vi "fWrite Binary.vi"(8 "error in":errorcluster, 9 "Samples per data chunk":u32, 10 "array":i16[](array[numeric]), 11 "refnum in":refnum<file>) -> (0 "error out":errorcluster, 3 "refnum out":refnum<file>, 5 "Data good?":bool)   [LabVIEW 2012]
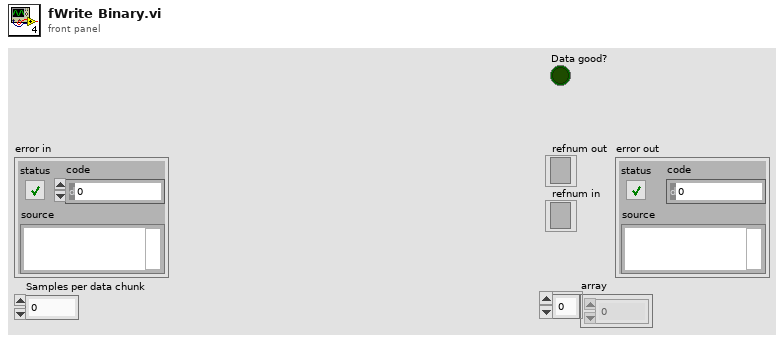
[diagram p1: front panel]
types:
  T1 = enum16{"big-endian, network order", "native, host order", "little-endian"}
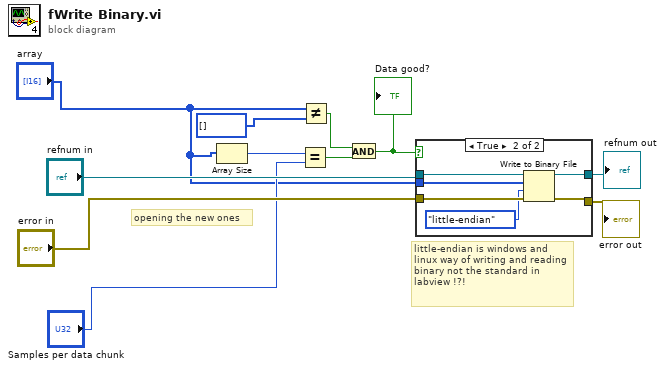
[diagram p0: block diagram]
diagram:
  # "little-endian is windows and linux way of writing and reading binary not the standard in labview !?!"
  # "opening the new ones"
  n1 = Array Size(array="array") -> (size(s)=w9:i32)
  n2 = Equal?(x=w9, y="Samples per data chunk") -> (x = y?=w8:bool)
  n3 = Not Equal?(x="array", y=i16[] []) -> (x != y?=w10:bool)
  n4 = And(x=w10, y=w8) -> (x .and. y?=w7:bool)
  "Data good?" <- w7
  n5 = case shown="True" w7 {
    tunnel: "error in" -> [w12 w19]
    tunnel: "refnum in" -> [w13 w18]
    tunnel: [w13 w17] -> w6
    tunnel: [w12 w16] -> w3
    tunnel: "array" -> [_ w15]
    frame False {
    }
    frame True {
      n6 = Write to Binary File(file (use dialog)=w18, data=w15, error in=w19, 9:T1."little-endian" ("byte order (0:big-endian, network order)")) -> (refnum out=w17:refnum<file>, error out=w16:errorcluster)  [unwired: 2 in, 1 out]
    }
  }
  "refnum out" <- w6
  "error out" <- w3
